vi "AlliGator New NLSF Parameter Map Resolution.vi"(9 "Is Full Image Parameter Map":bool, 10 "Old NLSF Parameters Map Y Resolution":i32, 11 "Old NLSF Parameters Map X Resolution":i32) -> (2 "New NLSF Parameters Map X Resolution":i32, 3 "New NLSF Parameters Map X Resolution":i32)   [LabVIEW 2021, in "AlliGator Decay Fit Parameter Map.lvlib"]
doc: "Map resolution conversion.\n\nIf <B>Is Full Image Parameter Map</B> is true, returns the input resolution parameters.\n\nIf not, returns -1."
uses:
  AlliGator Decay Fit Parameter Map.lvlib
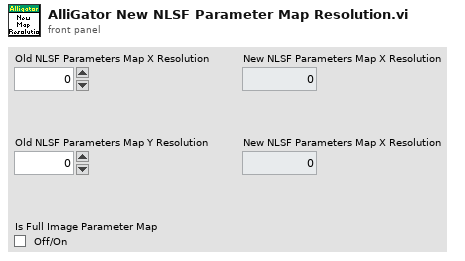
[diagram p1: front panel]
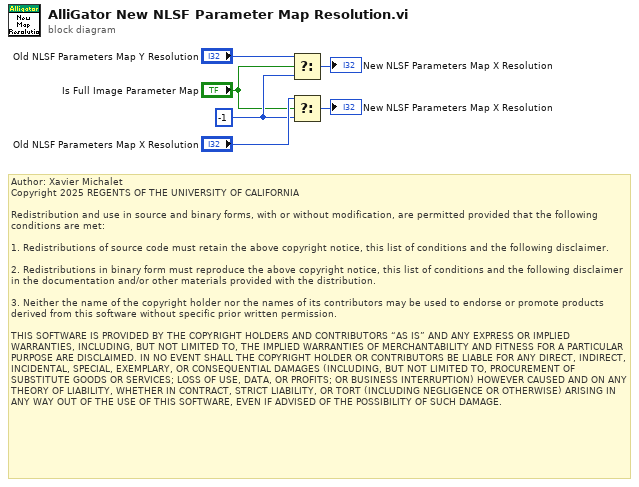
[diagram p0: block diagram]
diagram:
  w2 = -1 ("f")
  # "Author: Xavier Michalet\nCopyright 2025 REGENTS OF THE UNIVERSITY OF CALIFORNIA\n\nRedistribution and use in source and binary forms, with or without modification, are permitted provided that the following conditions are met:\n\n1. Redistributions of source code must retain the above copyright notice, this list of conditions and the following disclaimer.\n\n2. Redistributions in binary form must reproduce the above copyright notice, this list of conditions and the following disclaimer in the documentation and/or other materials provided with the distribution.\n\n3. Neither the name of the copyright holder nor the names of its contributors may be used to endorse or promote products derived from this software without specific prior written permission.\n\nTHIS SOFTWARE IS PROVIDED BY THE COPYRIGHT HOLDERS AND CONTRIBUTORS “AS IS” AND ANY EXPRESS OR IMPLIED WARRANTIES, INCLUDING, BUT NOT LIMITED TO, THE IMPLIED WARRANTIES OF MERCHANTABILITY AND FITNESS FOR A PARTICULAR PURPOSE ARE DISCLAIMED. IN NO EVENT SHALL THE COPYRIGHT HOLDER OR CONTRIBUTORS BE LIABLE FOR ANY DIRECT, INDIRECT, INCIDENTAL, SPECIAL, EXEMPLARY, OR CONSEQUENTIAL DAMAGES (INCLUDING, BUT NOT LIMITED TO, PROCUREMENT OF SUBSTITUTE GOODS OR SERVICES; LOSS OF USE, DATA, OR PROFITS; OR BUSINESS INTERRUPTION) HOWEVER CAUSED AND ON ANY THEORY OF LIABILITY, WHETHER IN CONTRACT, STRICT LIABILITY, OR TORT (INCLUDING NEGLIGENCE OR OTHERWISE) ARISING IN ANY WAY OUT OF THE USE OF THIS SOFTWARE, EVEN IF ADVISED OF THE POSSIBILITY OF SUCH DAMAGE."
  n1 = Select(t="Old NLSF Parameters Map Y Resolution", s="Is Full Image Parameter Map", f=w2) -> (s? t:f=→"New NLSF Parameters Map X Resolution":i32)
  n2 = Select(t="Old NLSF Parameters Map X Resolution", s="Is Full Image Parameter Map", f=w2) -> (s? t:f=→"New NLSF Parameters Map X Resolution":i32)
